vi "build-windows-flow.vi"(8 "error in":errorcluster, 10 "Delay [s]":u32, 11 "Operation":T3(ring)) -> (0 "error out":errorcluster, 3 "steps out":variant[](array[variant]))   [LabVIEW 2024]
uses:
  controls/UiStepBuilder.ctl
  controls/type.step-builder.ctl
  controls/state-engine.ctl
  controls/type.eng-call.proc-insert.ctl
  build.flowToVarient.vi
  Polymorphics/variantCtrl.polymorphic.vi
  Polymorphics/variantCtrlStepFunction.vi
  Polymorphics/variantCtrlSetpoint.vi
  Polymorphics/variantCtrlString.vi
  proc.util.enumToStrStepVar.vi
  util.DelimitedStringFromArray.vi
  Polymorphics/variantCtrlNumber.vi
  util.DelimitedStringToArray.vi
  proc.util.validateParamExist.vi
  <vilib>/Utility/error.llb/Clear Errors.vi
  <vilib>/Utility/error.llb/Trim Whitespace.vi
  <vilib>/Utility/error.llb/Trim Whitespace One-Sided.vi
  build.elementToParamString.vi
  util.error.create.vi
  Polymorphics/variantCtrlStepPointer.vi
  Polymorphics/variantCtrlStepUserMessage.vi
  Polymorphics/variantCtrlStepPath.vi
  globals/globals-engine.vi
panel:
  out "ProcName":string
  out "appended array":T1[](array[typedef])
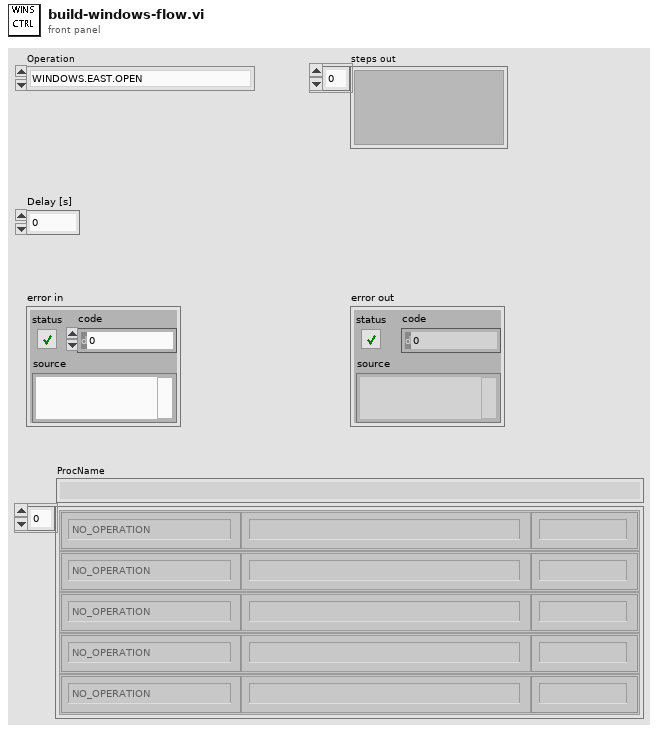
[diagram p1: front panel]
types:
  T1 = typedef "UiStepBuilder.ctl" = cluster{"Step Function":T2, "ParamString":string, "Step Label":string}
  T2 = typedef "type.step-builder.ctl" = enum16{"NO_OPERATION", "DELAY-JUMP", "DELAY", "JUMP", "COMPLETE", "SCHEDULER", "IRR-CHECK", "UNIT-CHECK", "UNIT-SAMPLE", "UNIT-DOSE", "LOG-REPORT", "LOG-MESSAGE", "IO-READ", "IO-READ-MANY", "IO-WRITE", "IO-COMPARE-OUT", "IO-COMPARE-IN", "PROC-START", "PROC-STOP", "PROC-LOAD", "PROC-IS-COMPLETED", "RECORD-MOVE", "GET-RH", "GET-UV", "GET-WD", "GET-WS", "OCS-CHECK", "OCS-RECORD"}
  T3 = enum16{"WINDOWS.EAST.OPEN", "WINDOWS.EAST.CLOSE", "WINDOWS.WEST.OPEN", "WINDOWS.WEST.CLOSE"}
  T4 = typedef "type.eng-call.proc-insert.ctl" = cluster{"ProcName":string, "instructions":variant[]}
  T5 = typedef "state-engine.ctl" = enum16{"ENG.NO-OP", "ENG.START", "ENG.STOP", "ENG.EXECUTE", "ENG.STATUS", "ENG.EXTERNAL-CALL", "ENG.INIT", "ENG.INIT.VARS", "ENG.INIT.SERIAL", "ENG.LOAD", "ENG.LOAD.SINGLE", "ENG.LOAD.MODULE", "ENG.LOAD.RELOAD", "ENG.LOAD.UNLOAD", "ENG.IO.LOAD", "ENG.IO.SAVE", "ENG.PROC.RELOAD-BY-NAME", "ENG.PROC.START", "ENG.PROC.STOP", "ENG.PROC.INSERT-STEPS", "ENG.PROC.ISRUNNING", "ENG.PROC.PRESET", "ENG.PROC.STATUS", "ENG.PRINT-USER-MSG", "ENG.RIO.SNAPSHOT", "ENG.RIO.AIN-SNAPSHOT-CALIB", "ENG.RIO.DOUT-BY-ADDR", "ENG.RIO.DOUT-BY-NAME", "ENG.RIO.RFS-DELAY-SET-X1", "ENG.RIO.RFS-DELAY-SET-X8", "ENG.RIO.RFS-CYCLES-SET", "ENG.RIO.RFS-CYCLES-GET", "ENG.RIO.RFS-ENABLE", "ENG.EXIT"}
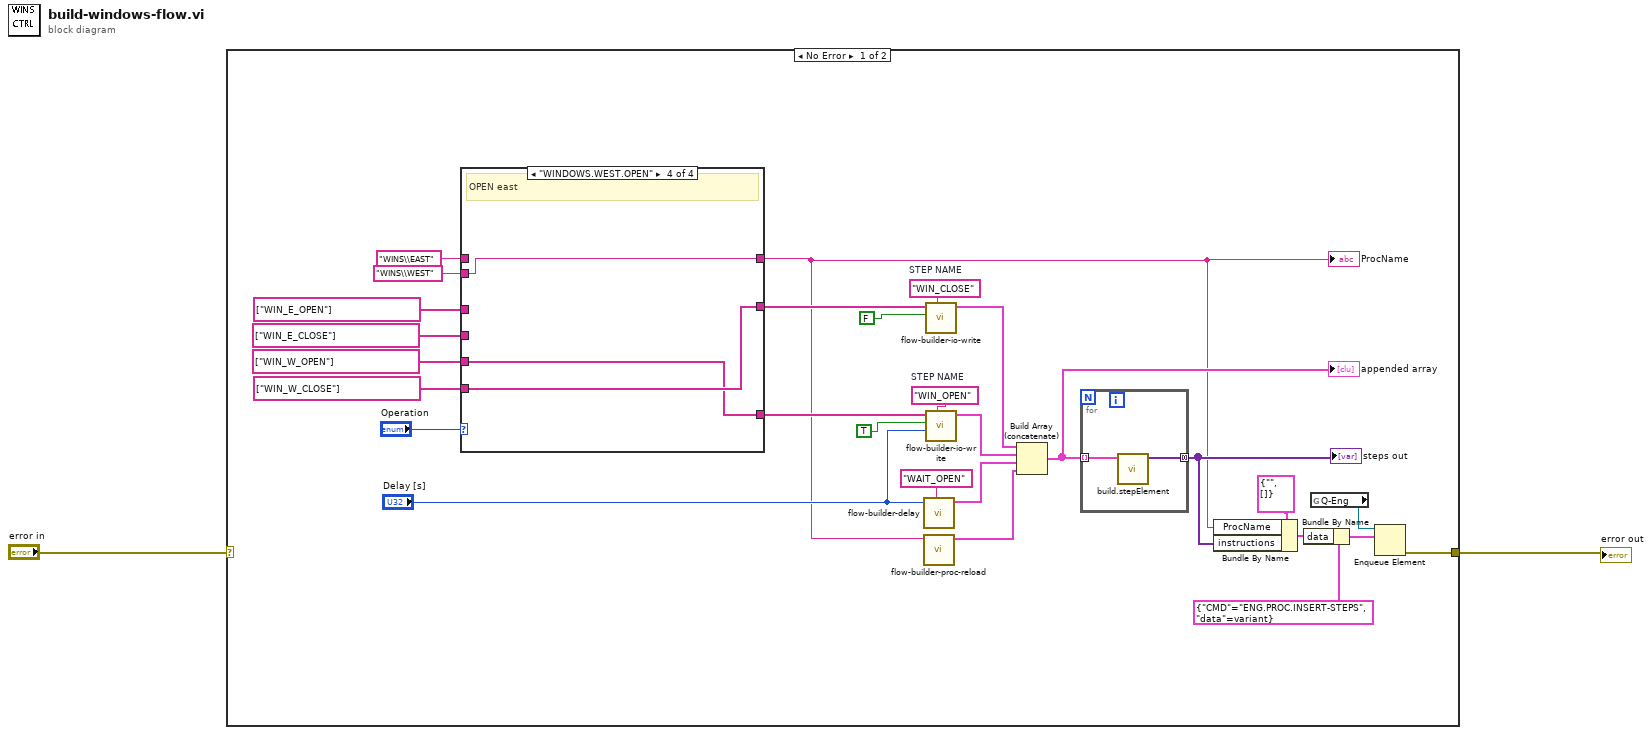
[diagram p0: block diagram]
diagram:
  n1 = case shown="No Error" "error in" {
    selector: "error in" -> [_ w45]
    tunnel: [w3 w45] -> w1
    frame No Error {
      w24 = "WIN_CLOSE"  # STEP NAME
      w26 = "WIN_OPEN"  # STEP NAME
      n2 = case shown="\"WINDOWS.WEST.OPEN\"" "Operation" {
        tunnel: [w31 w34 w37 w40] -> w25
        tunnel: [w32 w35 w38 w41] -> w22
        tunnel: "WINS\\WEST" ("ProcName") -> [_ _ w39 w42]
        tunnel: "WINS\\EAST" ("ProcName") -> [w33 w36 _ _]
        tunnel: [w33 w36 w39 w42] -> w8
        tunnel: string[] ["WIN_E_OPEN"] ("Dout+AUX") -> [w31 w35 _ _]
        tunnel: string[] ["WIN_E_CLOSE"] ("Dout+AUX") -> [w32 w34 _ _]
        tunnel: string[] ["WIN_W_OPEN"] ("Dout+AUX") -> [_ _ w38 w40]
        tunnel: string[] ["WIN_W_CLOSE"] ("Dout+AUX") -> [_ _ w37 w41]
        frame "WINDOWS.EAST.OPEN" {
          # "open east"
        }
        frame "WINDOWS.EAST.CLOSE" {
          # "CLOSE east"
        }
        frame "WINDOWS.WEST.CLOSE" {
          # "CLOSE east"
        }
        frame "WINDOWS.WEST.OPEN" {
          # "OPEN east"
        }
      }
      "ProcName" <- w8
      n3 = call "flow-builder-delay.vi"("Step Label"="WAIT_OPEN", "Delay [s]"="Delay [s]") -> ("Step Element"=w30:T1)  [unwired: 9 in]
      n4 = call "flow-builder-proc-reload.vi"("ProcPtr"=w8) -> ("Step Element"=w9:T1)  [unwired: 10 in]
      n5 = call "flow-builder-io-write.vi"("Step Name"=w24, "Value in"=FALSE ("UiDeviceConstant"), "Dout+AUX"=w22) -> ("Flow out"=w21:T1[])  [unwired: 8 in]
      n6 = call "flow-builder-io-write.vi"("Step Name"=w26, "Digital Timeout"="Delay [s]", "Value in"=TRUE ("UiDeviceConstant"), "Dout+AUX"=w25) -> ("Flow out"=w28:T1[])  [unwired: 7 in]
      n7 = Build Array (concatenate)(w21, w28, w30, w9) -> (w11:T1[])
      "appended array" <- w11
      n8 = for {
        tunnel: w11 -> [w44] mode=indexing
        tunnel: [w43] -> w14 mode=concatenating
        n9 = call "build.stepElement.vi"("Step in"=w44) -> ("steps out"=w43:variant[])  [unwired: 9 in, 1 out]
      }
      "steps out" <- w14
      n10 = Bundle By Name(cluster=T4 {"ProcName"="", "instructions"=[]}, "ProcName"=w8, "instructions"=w14) -> (w17:T4)
      n11 = Bundle By Name(cluster=cluster{"CMD":T5, "data":variant} {"CMD"=enum."ENG.PROC.INSERT-STEPS", "data"=variant} ("element"), "data"=w17) -> (w18:cluster{"CMD":T5, "data":variant})
      n12 = global read "globals-engine.vi" "Q-Eng"() -> (w19:refnum<queue>)
      n13 = Enqueue Element(queue=w19, element=w18) -> (error out=w3:errorcluster)  [unwired: 2 in, 2 out]
    }
    frame Error {
    }
  }
  "error out" <- w1
